vi "ExtractData.vi"(8 "Samples per freq calc":dbl=10000.0, 11 "Data input":waveform(dbl)[](array[waveform])) -> (3 "Data cluster":T1)   [LabVIEW 2019]
uses:
  <vilib>/measure/madcrms.llb/Basic Averaged DC-RMS for 1 Chan.vi
  <vilib>/gmath/NI_Gmath.lvlib
  <vilib>/measure/NI_MAPro.lvlib
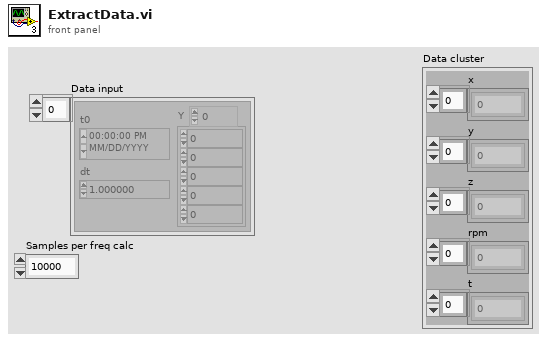
[diagram p1: front panel]
types:
  T1 = cluster{"x":dbl[], "y":dbl[], "z":dbl[], "rpm":dbl[], "t":dbl[]}
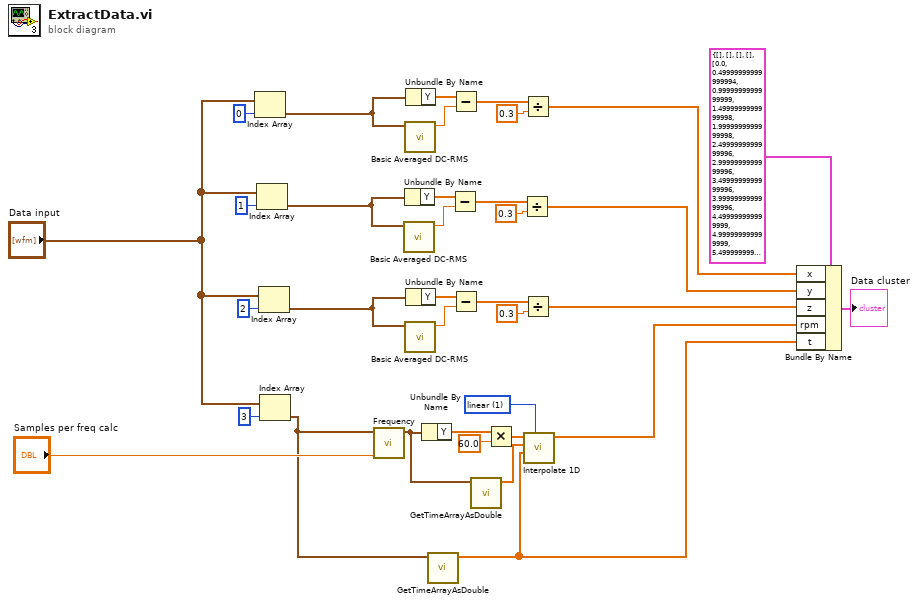
[diagram p0: block diagram]
diagram:
  w30 = 1 items=["nearest", "linear", "spline", "cubic Hermite", "Lagrange"] ("method")
  n1 = Index Array(array="Data input", index=0) -> (element=w7:waveform(dbl))
  n2 = Index Array(array="Data input", index=1) -> (element=w8:waveform(dbl))
  n3 = Index Array(array="Data input", index=2) -> (element=w9:waveform(dbl))
  n4 = Index Array(array="Data input", index=3) -> (element=w6:waveform(dbl))
  n5 = call "Frequency.vi"("Samples per calculation"="Samples per freq calc", "Input waveform"=w6) -> ("Frequency waveform"=w31:waveform(dbl))  [unwired: 9 in]
  n6 = call-poly <vilib>:"Basic Averaged DC-RMS.vi"("signal in"=w8) -> ("DC value"=w22:dbl)  [unwired: 7 in, 3 out]
  n7 = call-poly <vilib>:"Basic Averaged DC-RMS.vi"("signal in"=w7) -> ("DC value"=w26:dbl)  [unwired: 7 in, 3 out]
  n8 = Unbundle By Name(w8) -> ("Y"=w23:dbl[])
  n9 = call-poly <vilib>:"Basic Averaged DC-RMS.vi"("signal in"=w9) -> ("DC value"=w18:dbl)  [unwired: 7 in, 3 out]
  n10 = Unbundle By Name(w7) -> ("Y"=w27:dbl[])
  n11 = Unbundle By Name(w9) -> ("Y"=w19:dbl[])
  n12 = Unbundle By Name(w31) -> ("Y"=w35:dbl[])
  n13 = call "GetTimeArrayAsDouble.vi"("Waveform"=w6) -> ("Time Array"=w10:dbl[])  [unwired: 10 in]
  n14 = Subtract(x=w23, y=w22) -> (x-y=w24:dbl[])
  n15 = Subtract(x=w27, y=w26) -> (x-y=w28:dbl[])
  n16 = Subtract(x=w19, y=w18) -> (x-y=w20:dbl[])
  n17 = call "GetTimeArrayAsDouble.vi"("Waveform"=w31) -> ("Time Array"=w32:dbl[])  [unwired: 10 in]
  n18 = Multiply(x=w35, y=60.0) -> (x*y=w33:dbl[])
  n19 = Divide(x=w24, y=0.3) -> (x/y=w4:dbl[])
  n20 = Divide(x=w28, y=0.3) -> (x/y=w3:dbl[])
  n21 = Divide(x=w20, y=0.3) -> (x/y=w5:dbl[])
  n22 = call <vilib>:"Interpolate 1D.vi"("method"=w30, "xi"=w10, "X"=w32, "Y"=w33) -> ("yi"=w11:dbl[])  [unwired: 5 in, 2 out]
  n23 = Bundle By Name(cluster=T1 {"x"=[], "y"=[], "z"=[], "rpm"=[], "t"=[0.0, 0.49999999999999994, 0.9999999999999999, 1.4999999999999998, 1.9999999999999998, 2.4999999999999996, 2.9999999999999996, 3.4999999999999996, 3.9999999999999996, 4.499999999999999, 4.999999999999999, 5.499999999999999, 5.999999999999999, 6.499999999999999, 6.999999999999999, 7.499999999999999, 7.999999999999999, 8.499999999999998, 8.999999999999998, 9.499999999999998, 9.999999999999998, 10.499999999999998, 10.999999999999998, 11.499999999999998, 11.999999999999998, 12.499999999999998, 12.999999999999998, 13.499999999999998, 13.999999999999998, 14.499999999999998, 14.999999999999998, 15.499999999999998, 15.999999999999998, 16.499999999999996]} ("input cluster"), "x"=w3, "y"=w4, "z"=w5, "rpm"=w11, "t"=w10) -> (→"Data cluster":T1)
